vi "Start Async.vi"(9 "Queue Caller":map{string, refnum<data-value>}(c390), 10 "Queue of Queue Self":refnum<queue>, 11 "Queue Actor":refnum<class "Queue Actor.lvclass">) -> (0 "error out":errorcluster)   [LabVIEW 2021, in "jettl Queue Actor.lvlib" / "jettl Queue Actor.lvclass"]
uses:
  jettl Queue Actor.lvclass
  Actor/Msg/Msg.lvclass
  Actor/Queue Actor/Queue Actor.lvclass
  Queue Actor.vi
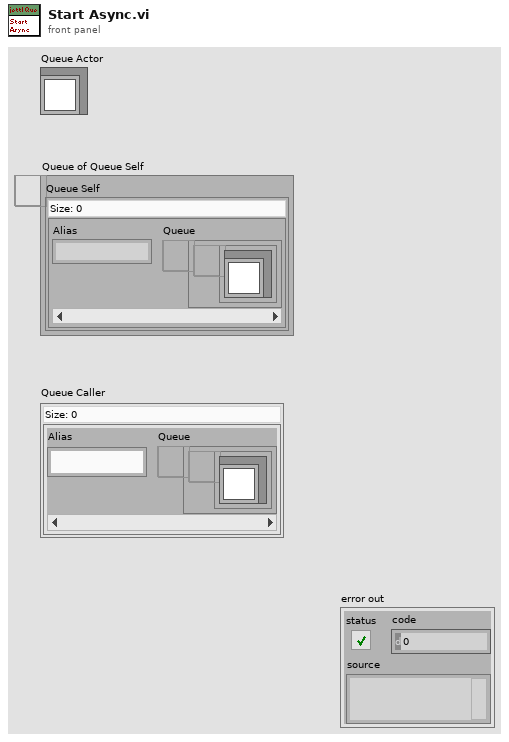
[diagram p1: front panel]
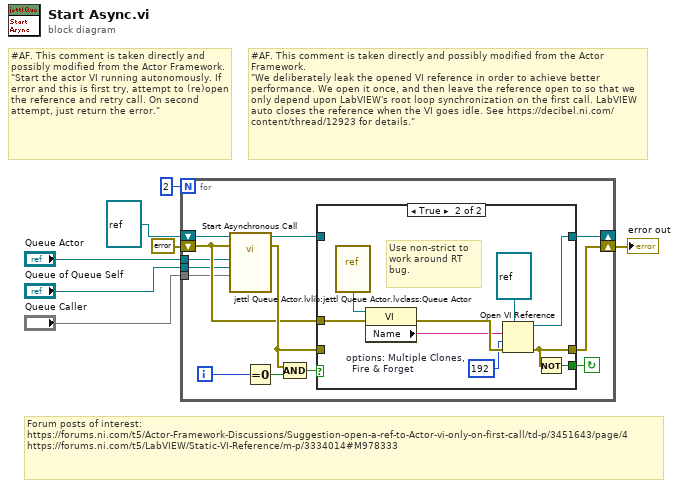
[diagram p0: block diagram]
diagram:
  # "Forum posts of interest:\nhttps://forums.ni.com/t5/Actor-Framework-Discussions/Suggestion-open-a-ref-to-Actor-vi-only-on-first-call/td-p/3451643/page/4\nhttps://forums.ni.com/t5/LabVIEW/Static-VI-Reference/m-p/3334014#M978333"
  # "#AF. This comment is taken directly and possibly modified from the Actor Framework.\n\"We deliberately leak the opened VI reference in order to achieve better performance. We open it once, and then leave the reference open to so that we only depend upon LabVIEW's root loop synchronization on the first call. LabVIEW auto closes the reference when the VI goes idle. See https://decibel.ni.com/content/thread/12923 for details.\""
  # "#AF. This comment is taken directly and possibly modified from the Actor Framework.\n\"Start the actor VI running autonomously. If error and this is first try, attempt to (re)open the reference and retry call. On second attempt, just return the error.\""
  n1 = for {
    N: 2 -> [_]
    shift-right: [w20] -> _
    shift-left: refnum<vi> refnum -> [w19]
    shift-right: [w17] -> w5
    shift-left: errorcluster {"status"=FALSE, "code"=0, "source"=""} ("error out") -> [w11]
    tunnel: "Queue Actor" -> [w10]
    tunnel: "Queue Caller" -> [w8]
    tunnel: "Queue of Queue Self" -> [w9]
    i -> [w14]
    stop <- w12 continue-if-true
    n2 = call-by-ref "Start Asynchronous Call"(reference=w19, error in=w11, "Queue Caller"=w8, "Queue of Queue Self"=w9, "Queue Actor"=w10) -> (reference out=w18:refnum<vi>, error out=w13:errorcluster)  [unwired: 9 in]
    n3 = Equal To 0?(x=w14) -> (x = 0?=w15:bool)
    n4 = Compound Arithmetic op=AND(w13, w15) -> (w16:bool)
    n5 = case shown="True" w16 {
      tunnel: [w22 w28] -> w20
      tunnel: [w21 w26] -> w17
      tunnel: w18 -> [w22 _]
      tunnel: w13 -> [w21 _]
      tunnel: [_ w27] -> w12
      tunnel: w11 -> [_ w25]
      frame False {
      }
      frame True {
        w29 = 192  # options: Multiple Clones,   Fire & Forget
        # "Use non-strict to work around RT bug."
        n6 = vi-ref "jettl Queue Actor.lvlib:jettl Queue Actor.lvclass:Queue Actor.vi"() -> (w24:refnum<vi>)
        n7 = property class="VI"(reference=w24, error in=w25) -> (error out=w31:errorcluster, "Name"=w30:string)  [unwired: 1 out]
        n8 = Open VI Reference(type specifier VI Refnum (for type only)=refnum<vi> refnum, vi path=w30, options=w29, error in (no error)=w31) -> (vi reference=w28:refnum<vi>, error out=w26:errorcluster)  [unwired: 2 in]
        n9 = Not(x=w26) -> (.not. x?=w27:bool)
      }
    }
  }
  "error out" <- w5
